vi "FFT.vi"(2 "TransformType":enum16{"Normal FFT", "Inverse FFT"}(ring), 5 "Complex Input Data":cdb[](array[numeric]) format="%.2f") -> (0 "DLL Return Code":i32, 1 "complex FFT":cdb[](array[numeric]) format="%.2f")   [LabVIEW 2012]
uses:
  LtMath.dll
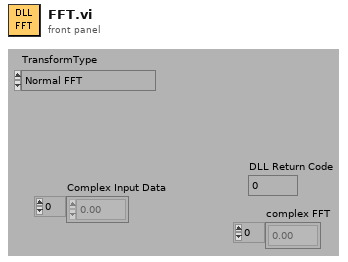
[diagram p1: front panel]
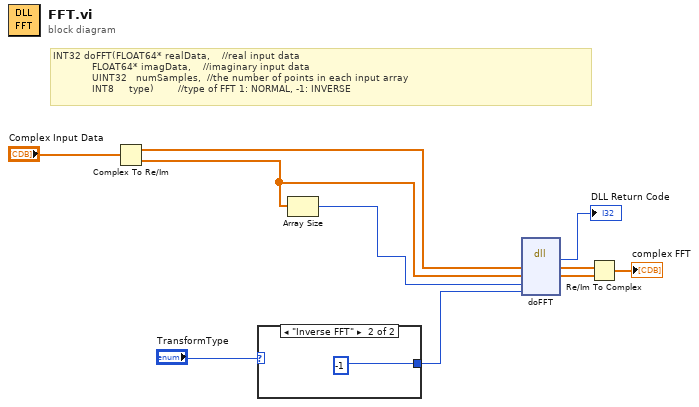
[diagram p0: block diagram]
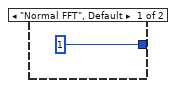
[diagram p2: hidden frame]
diagram:
  # "INT32 doFFT(FLOAT64* realData,    //real input data\n             FLOAT64* imagData,    //imaginary input data\n             UINT32   numSamples,  //the number of points in each input array\n             INT8     type)        //type of FFT 1: NORMAL, -1: INVERSE"
  n1 = Complex To Re/Im(x + iy="Complex Input Data") -> (x=w2:dbl[], y=w1:dbl[])
  n2 = case shown="\"Inverse FFT\"" "TransformType" {
    tunnel: [i8 1 i8 -1] -> w9
    frame "Normal FFT", Default {
    }
    frame "Inverse FFT" {
    }
  }
  n3 = Array Size(array=w1) -> (size(s)=w4:i32)
  n4 = dll-call lib="LtMath.dll" fn="doFFT"("realData"=w2, "imagData"=w1, "numSamples"=w4, "type"=w9) -> ("return type"=→"DLL Return Code":i32, "realData"=w8:dbl[], "imagData"=w7:dbl[])  [unwired: 5 in, 2 out]
  n5 = Re/Im To Complex(1:w7, 2:w8) -> (0:→"complex FFT":cdb[])
